vi "Sienar Band - Main Panel.vi"() -> ()   [LabVIEW 2016]
uses:
  <userlib>/LVLibSVM/LibSVM Sparse/Controls/Grid parameters.ctl
  <vilib>/Math Plots/3D Math Plots/3D Surface/3D Surface XCtrl/3D Surface.xctl
  Typedef/SVM predict class.ctl
  Typedef/SVM train class.ctl
  Typedef/SIENAR Band - States.ctl
  <vilib>/BLE/type_def/connection_status_bundle.ctl
  <vilib>/BLE/type_def/address_type.ctl
  Typedef/Event cluster.ctl
  <userlib>/LVLibSVM/LibSVM Dense/Wrapper API/Controls/svmdense_problem.ctl
  <userlib>/LVLibSVM/LibSVM Dense/Wrapper API/Controls/svmdense_model.ctl
  <userlib>/LVLibSVM/LibSVM Sparse/Wrapper API/Controls/svm_parameter.ctl
  <userlib>/LVLibSVM/LibSVM Sparse/Wrapper API/Controls/svm_type.ctl
  <userlib>/LVLibSVM/LibSVM Sparse/Wrapper API/Controls/svm_kernel_type.ctl
  Typedef/BLE char handle.ctl
  <userlib>/LVLibSVM/LibSVM Sparse/Controls/Options Training.ctl
  <userlib>/LVLibSVM/LibSVM Dense/SubVIs/SVM Dense Train C_SVC.vi
  <userlib>/LVLibSVM/LibSVM Dense/Wrapper API/svmdense_predict.vi
  <userlib>/LVLibSVM/Tools/SubVIs/Dense - Scale Problem Linear.vi
  <userlib>/LVLibSVM/LibSVM Dense/Wrapper API/svmdense_train.vi
  <vilib>/Utility/xml.llb/Read From XML File(string).vi
  <vilib>/Utility/xml.llb/Write to XML File(string).vi
panel:
  in  "Show RAW data":bool
  in  "Tab Control":T1(tab)
  in  "Timeout":u16=1000 format="%.0fms"
  in  "Latency":u16 max=500 step=1
  in  "Max interval":u16=50 caption="Connection interval (max)" min=10 max=4000 step=1 format="%.0fms"
  in  "Min interval":u16=20 caption="Connection interval (min)" min=10 max=4000 step=1 format="%.0fms"
  out "Devices":i32(listbox)=-1
  out "BLE Status":bool
  in  "Connect BLE":bool
  in  "Address type":enum8{"Public", "Random"}(ring)
  in  "MAC Address":string="24:0A:C4:04:1C:4E"
  out "BLED112 Dongle Info":string
  in  "Connect dongle":bool
  out "Dongle Status":bool
  in  "USB BLE Dongle port":refnum<visa-resource-name>
  in  "Discover":bool
  in  "Notes":string
  in  "User name":string
  in  "Test label":string
  in  "Open MPU calib":bool
  in  "Acquisition interval":u32=50 min=50 max=1000 step=10 format="%.0fms"
  in  "MPU calib":path=path "C:/Users/Frax/Desktop/Sienar-Band/MPU_calib.ini" caption="Choose MPU calibration file:"
  in  "Confirm settings":bool
  out "Strain chart":T2(graph)
  in  "Open adv viewer":bool
  in  "Stream data":bool
  in  "Clear Plot":bool
  out "YPR chart":cluster{"Yaw":sgl, "Pitch":sgl, "Roll":sgl}(graph)
  in  "Save RAW data":bool
  in  "Open MPU panel":bool
  in  "Save SVM model":bool
  in  "Learn from data":bool
  in  "Split data":bool=TRUE caption="Split data set for cross-validation"
  in  "Load data set":bool
  in  "SVM train Class":T3
  in  "Append data":bool=TRUE caption="Append data to file"
  in  "Save Data set":bool
  in  "Train":bool
  out "Event Going on?":bool
  out "Event Count":u32
  out "Gridsearch result":refnum<class "3D Plot Datatype.lvclass">[](xcontrol)
  in  "Grid parameters":T4={"C start"=-5.0, "Gamma start"=-15.0, "C end"=15.0, "C step"=4.0, "K"=10, "Gamma end"=3.0, "Gamma step"=4.0, "random seed"=-1}
  out "Class detected":T5
  in  "Predict":bool
  in  "Load SVM model":bool
  in  "Exit":bool
  in  "Connection panel":bool
  in  "SVM Analysis panel":bool
  in  "SVM Train panel":bool
  in  "Settings panel":bool
  # "Acquisition settings"
  # "OR"
  # "User settings"
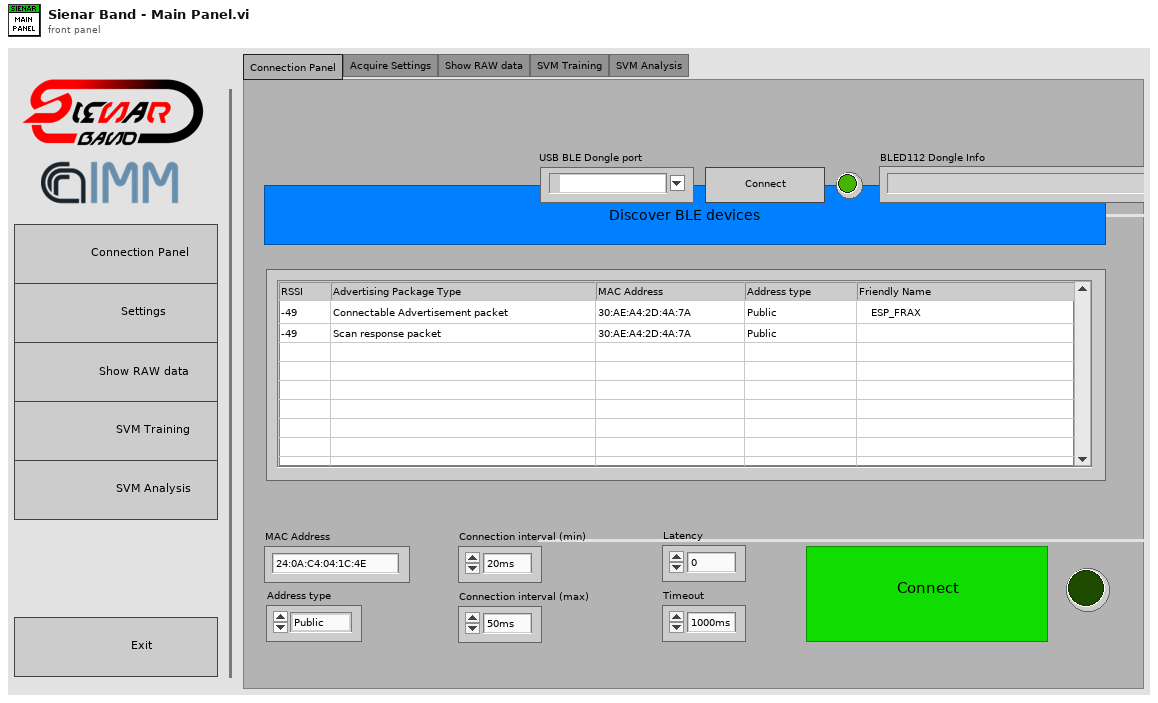
[diagram p1: front panel]
types:
  T1 = enum32{"Connection Panel", "Acquire Settings", "Show RAW data", "SVM Training", "SVM Analysis"}
  T2 = cluster{"Strain sensor 1":sgl, "Strain sensor 2":sgl, "Strain sensor 3":sgl, "Strain sensor 4":sgl, "Strain sensor 5":sgl, "Strain sensor 6":sgl, "Strain sensor 7":sgl, "Strain sensor 8":sgl}
  T3 = typedef "SVM train class.ctl" = enum16{"Grab/Grab release", "Hand flexion/HF release", "Hand extension/HE release", "Tap", "Swipe_CW", "Swipe_CCW"}
  T4 = typedef "Grid parameters.ctl" = cluster{"C start":dbl, "Gamma start":dbl, "C end":dbl, "C step":dbl, "K":i32, "Gamma end":dbl, "Gamma step":dbl, "random seed":i32}
  T5 = typedef "SVM predict class.ctl" = enum16{"Grab", "Grab release", "Hand flexion", "Hand flexion release", "Hand extension", "Hand extension release", "Tap", "Swipe_CW", "Swipe_CCW"}
  T6 = cluster{"Strain data":cluster{"Strain sensor 1":sgl, "Strain sensor 2":sgl, "Strain sensor 3":sgl, "Strain sensor 4":sgl, "Strain sensor 5":sgl, "Strain sensor 6":sgl, "Strain sensor 7":sgl, "Strain sensor 8":sgl}, "YPR data":cluster{"Yaw":sgl, "Pitch":sgl, "Roll":sgl}}
  T7 = typedef "connection_status_bundle.ctl" = cluster{"MAC Address":string, "cnx handle":u8, "cnx flags":u8, "Address Type":T8, "Connection Interval (ms)":u16, "Timeout(ms)":u16, "Latency":u16, "bonding handle":u8}
  T8 = typedef "address_type.ctl" = u8
  T9 = typedef "Event cluster.ctl" = cluster{"Base line":dbl[], "Event data":dbl[][], "Duration":dbl, "Event ongoing":bool, "SVM train Class":T3, "SVM predict Class":T5}
  T10 = typedef "svmdense_problem.ctl" = cluster{"Y":dbl[], "X":cluster{"x":dbl[]}[]}
  T11 = typedef "svmdense_model.ctl" = cluster{"param":T12, "nr_class":i32, "l":i32, "SV":cluster{"Array":dbl[]}[], "sv_coef":dbl[][], "rho":dbl[], "probA":dbl[], "probB":dbl[], "sv_indices":i32[], "label":i32[], "nSV":i32[]}
  T12 = typedef "svm_parameter.ctl" = cluster{"svm_type":T13, "kernel_type":T14, "degree":i32, "gamma":dbl, "coef0":dbl, "cache_size":dbl, "eps":dbl, "C":dbl, "weight_label":i32[], "weight":dbl[], "nu":dbl, "p":dbl, "shrinking":bool, "probability":bool}
  T13 = typedef "svm_type.ctl" = enum32{"C_SVC", "NU_SVC", "ONE_CLASS", "EPSILON_SVR", "NU_SVR"}
  T14 = typedef "svm_kernel_type.ctl" = enum32{"LINEAR", "POLY", "RBF", "SIGMOID", "PRECOMPUTED"}
  T15 = cluster{"Conn Status":T7, "MAC Address":string, "Is Connected":bool, "Handle table":string[][], "channel map":u16, "Event cluster":T9, "Data set":dbl[][], "Dense Problem":T10, "Model":T11}
  T16 = typedef "SIENAR Band - States.ctl" = enum16{"Idle", "Connect Dongle", "Discover BLE", "Connect BLE", "Discover Services", "Disconnect BLE", "Confirm settings", "Open advanced viewer", "Open MPU panel", "Set Stream settings", "Stream data", "Stop stream", "Stop", "Save RAW data", "SVM - Train", "SVM - Check for event", "SVM - Extract features", "SVM - Learn from data", "SVM - Load data set", "SVM - Save data set", "SVM - Load SVM model", "SVM - Save SVM model", "SVM - Start predict", "Exit"}
  T17 = typedef "Options Training.ctl" = cluster{"cache_size":dbl, "eps":dbl, "shrinking":bool, "probability":bool}
  T18 = enum16{"open", "replace", "create", "open or create", "replace or create", "replace or create with confirmation"}
  T19 = typedef "BLE char handle.ctl" = u16
  T20 = cluster{"Avg Strain data out":cluster{"Strain sensor 1":sgl, "Strain sensor 2":sgl, "Strain sensor 3":sgl, "Strain sensor 4":sgl, "Strain sensor 5":sgl, "Strain sensor 6":sgl, "Strain sensor 7":sgl, "Strain sensor 8":sgl}, "YPR data":cluster{"Yaw":sgl, "Pitch":sgl, "Roll":sgl}}
  T21 = cluster{"Strain sensor 1":sgl, "Strain sensor 2":sgl, "Strain sensor 3":sgl, "Strain sensor 4":sgl, "Strain sensor 5":sgl, "Strain sensor 6":sgl, "Strain sensor 7":sgl, "Strain sensor 8":sgl}[]
  T22 = typedef "Kernel.ctl" = cluster{"Type":T14, "Degree":i32, "Gamma":dbl, "Coef0":dbl}
  T23 = typedef "Parameters C_SVC.ctl" = cluster{"C":dbl, "weight_label":i32[], "weight":dbl[]}
  T24 = cluster{"libsvm options":T17, "libsvm weights":T23}
  T25 = typedef "svm_problem.ctl" = cluster{"y":dbl[], "x":cluster{T26[]}[]}
  T26 = typedef "svm_node.ctl" = cluster{"index":i32, "value":dbl}
  T27 = cluster{"Strain sensor 1":dbl, "Strain sensor 2":dbl, "Strain sensor 3":dbl, "Strain sensor 4":dbl, "Strain sensor 5":dbl, "Strain sensor 6":dbl, "Strain sensor 7":dbl, "Strain sensor 8":dbl}[]
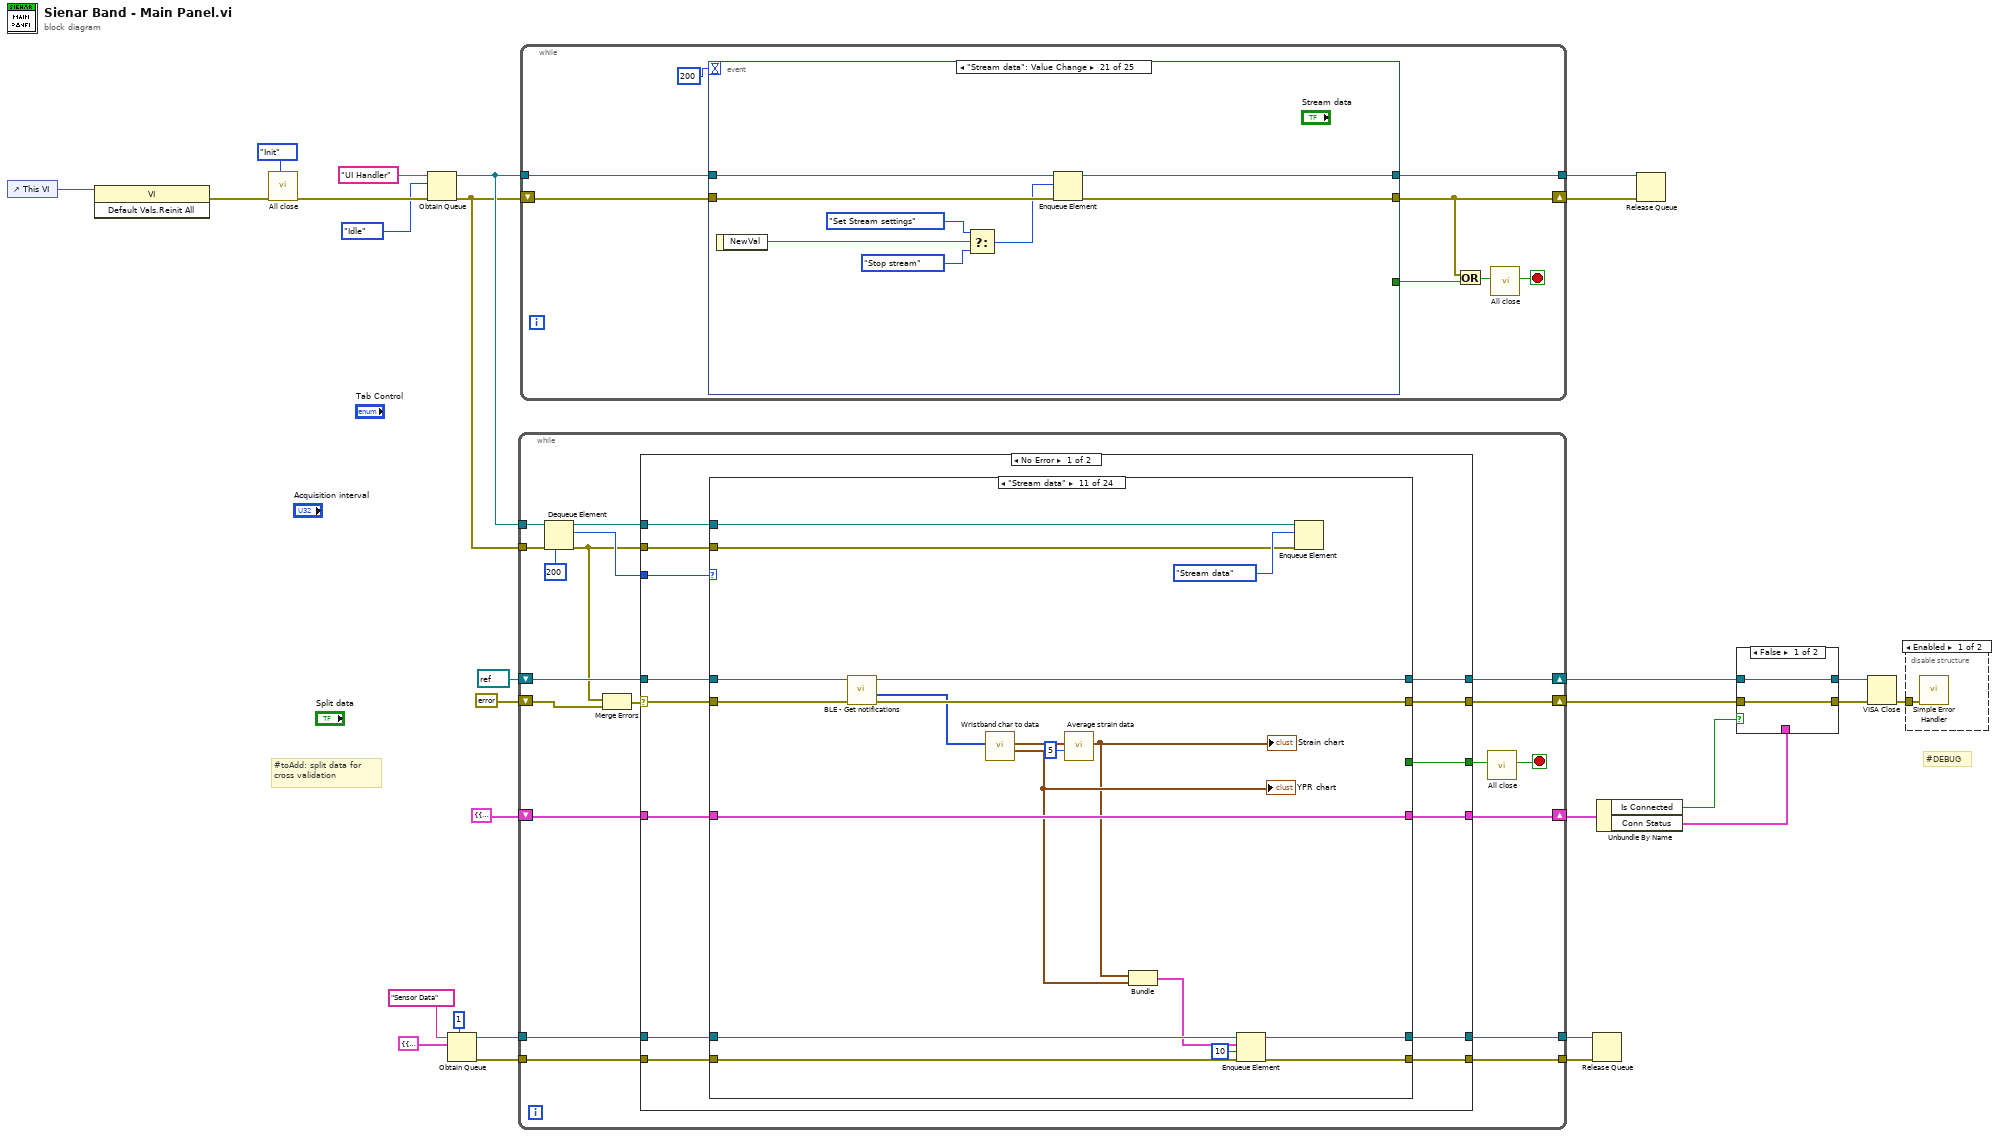
[diagram p0: block diagram]
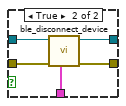
[diagram p3: hidden frame]
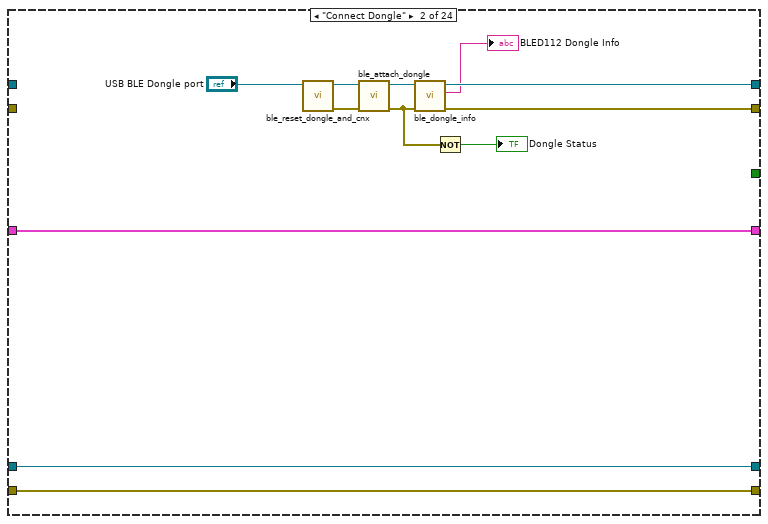
[diagram p5: hidden frame]
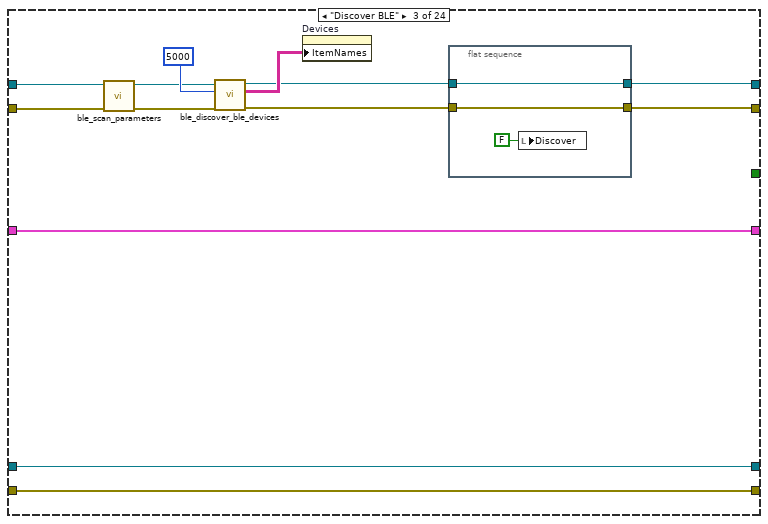
[diagram p6: hidden frame]
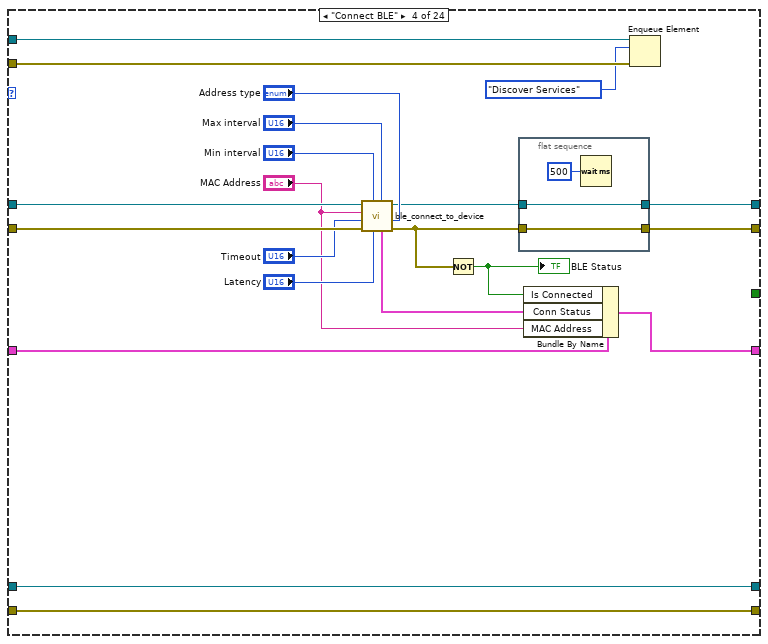
[diagram p7: hidden frame]
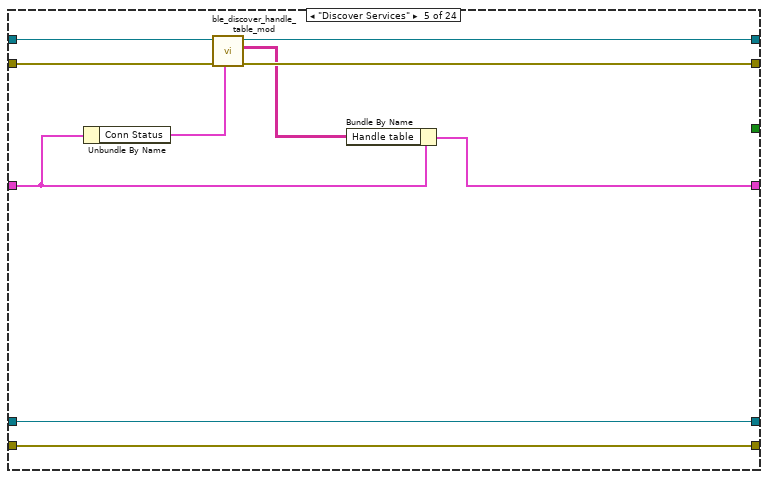
[diagram p8: hidden frame]
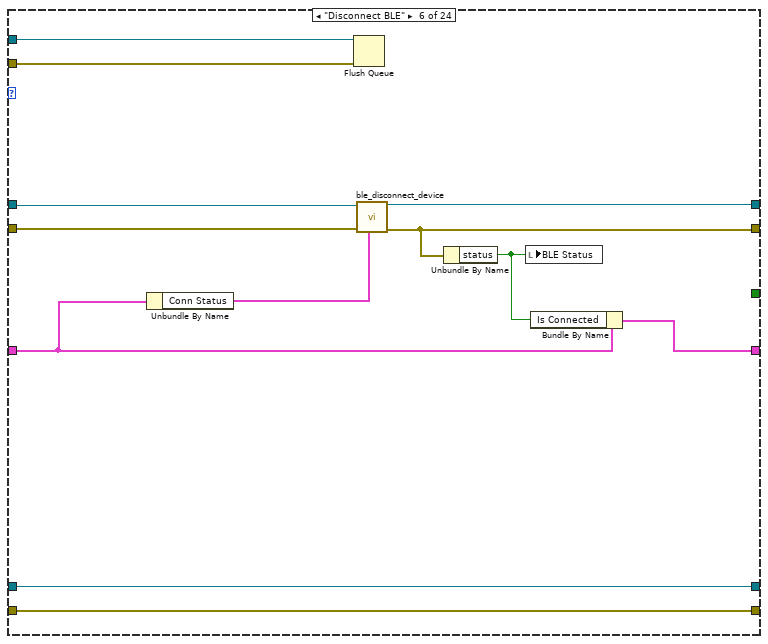
[diagram p9: hidden frame]
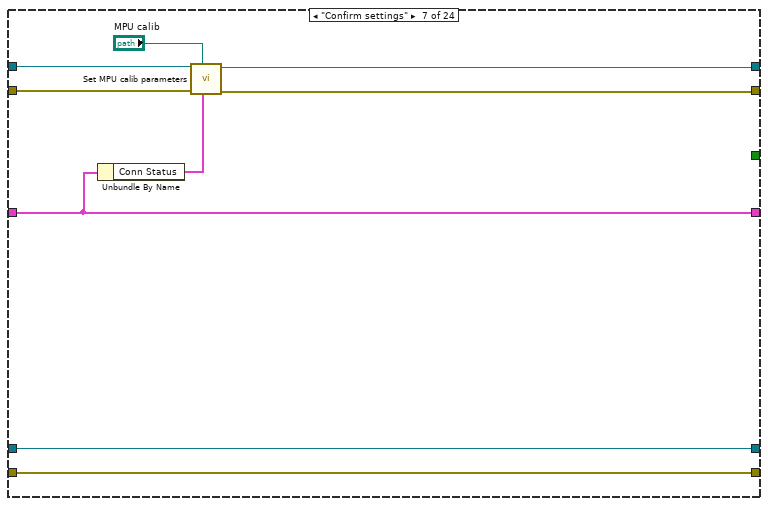
[diagram p10: hidden frame]
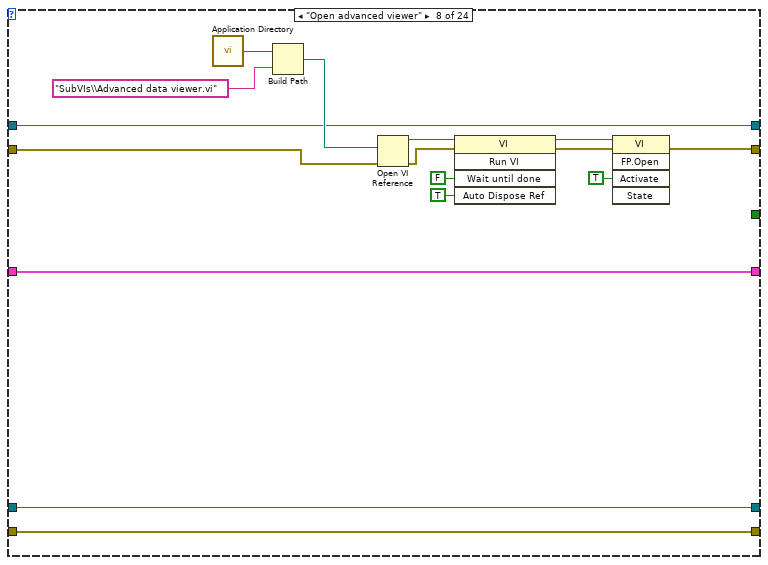
[diagram p11: hidden frame]
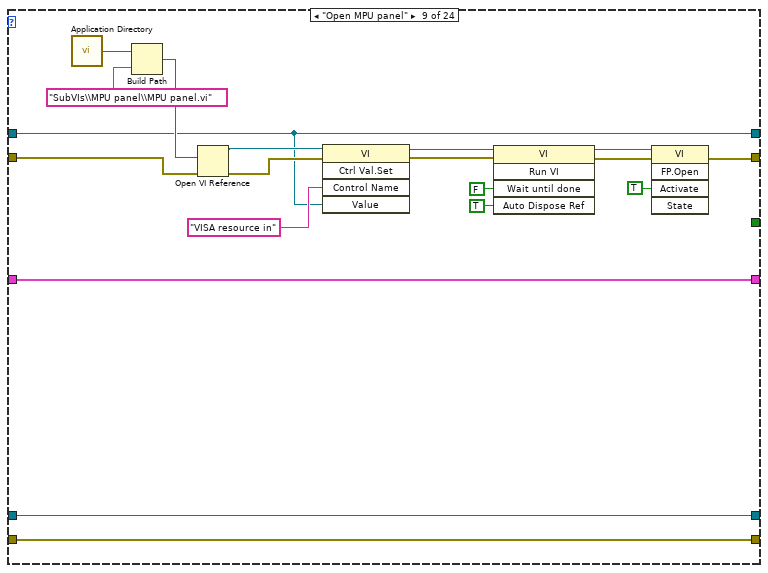
[diagram p12: hidden frame]
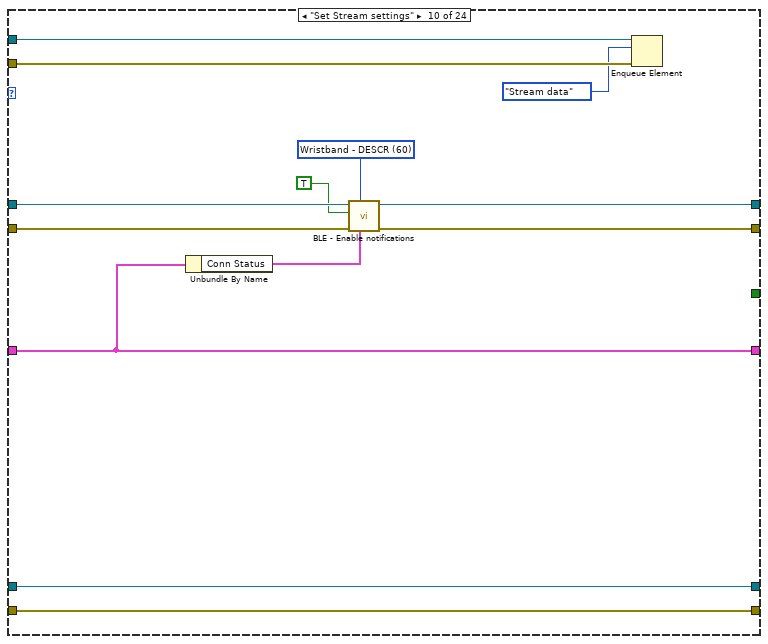
[diagram p13: hidden frame]
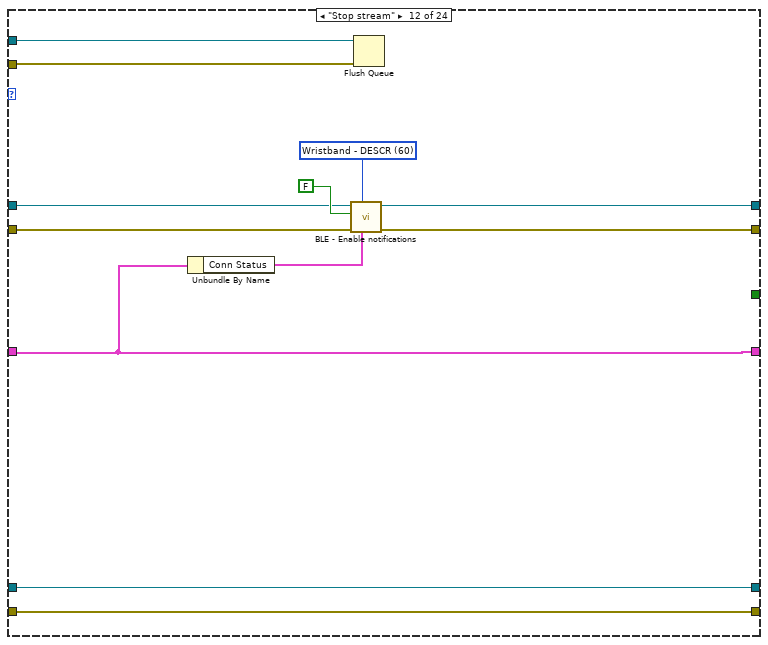
[diagram p14: hidden frame]
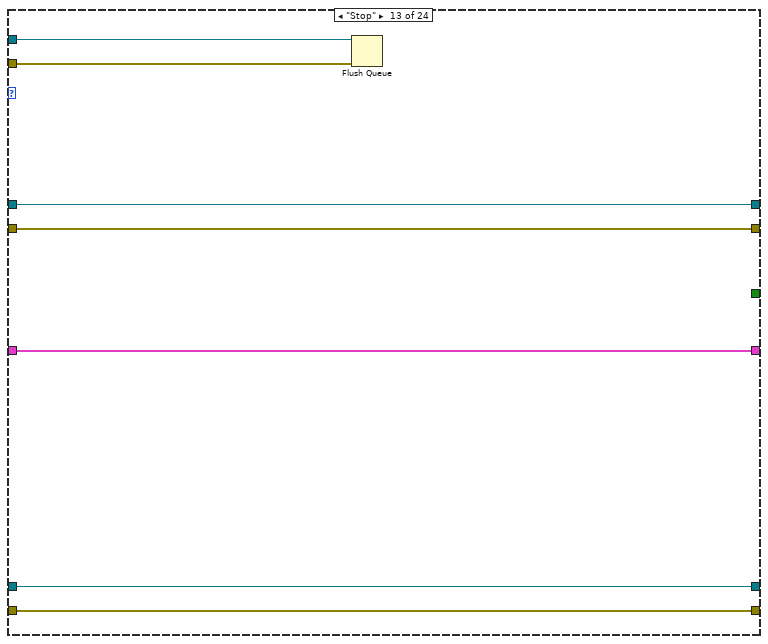
[diagram p15: hidden frame]
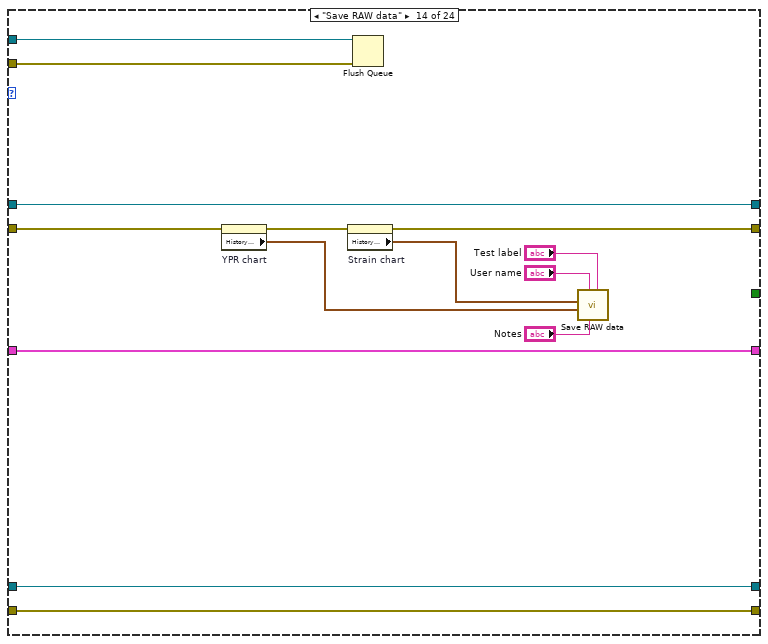
[diagram p16: hidden frame]
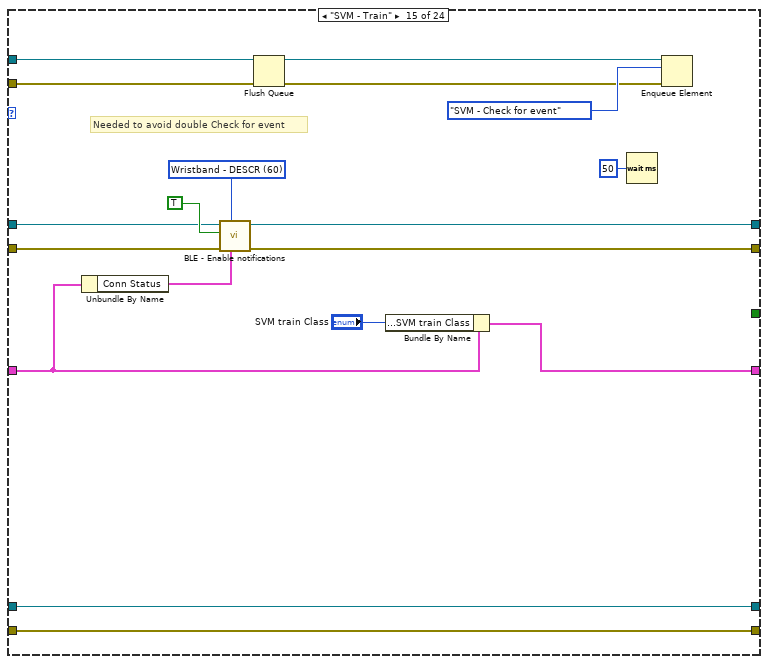
[diagram p17: hidden frame]
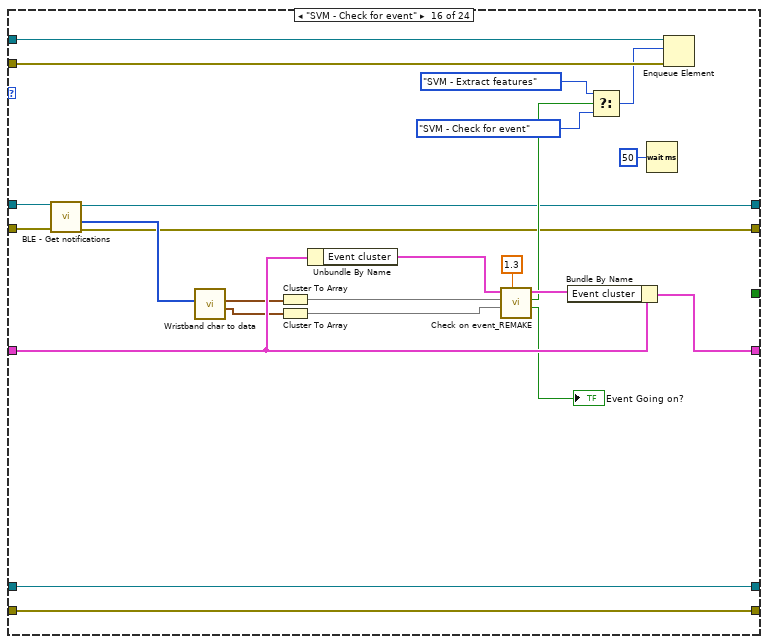
[diagram p18: hidden frame]
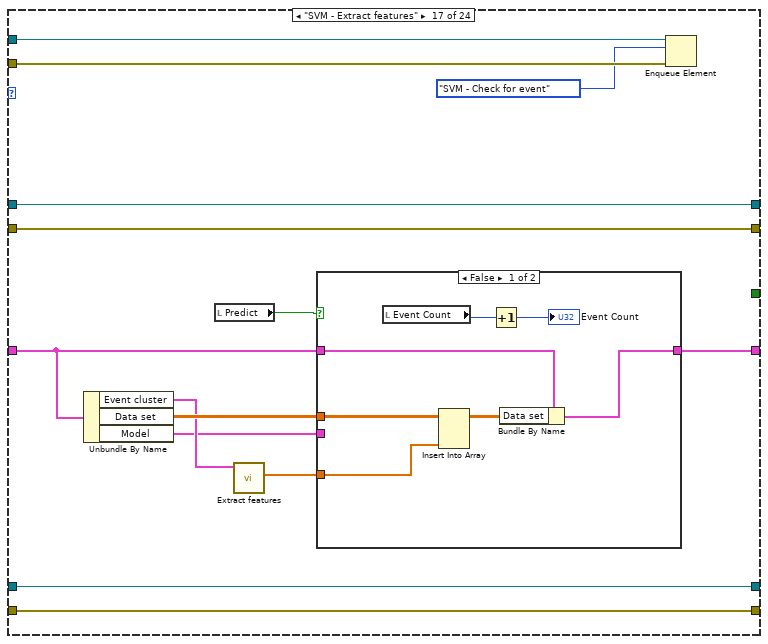
[diagram p19: hidden frame]
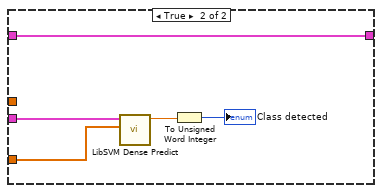
[diagram p20: hidden frame]
diagram:
  # "#toAdd: split data for\ncross validation"
  # "#DEBUG"
  n1 = control-ref of="This VI"() -> (w23:refnum<vi>)
  n2 = invoke class="VI" method="Default Vals.Reinit All"(reference=w23) -> (error out=w22:errorcluster)  [unwired: 2 in, 2 out]
  n3 = call "All close.vi"("Operation (Check)"=enum16{"Init", "Check"}."Init", "Error In"=w22) -> ("Error Out"=w25:errorcluster)  [unwired: 8 in, 1 out]
  n4 = Obtain Queue(name (unnamed)="UI Handler", element data type=SIENAR_Band_-_States."Idle", error in (no error)=w25) -> (queue out=w21:refnum<queue>, error out=w20:errorcluster)  [unwired: 2 in, 1 out]
  n5 = Obtain Queue(max queue size (-1, unlimited)=1, name (unnamed)="Sensor Data", element data type=T6 {"Strain data"={"Strain sensor 1"=0.0, "Strain sensor 2"=0.0, "Strain sensor 3"=0.0, "Strain sensor 4"=0.0, "Strain sensor 5"=0.0, "Strain sensor 6"=0.0, "Strain sensor 7"=0.0, "Strain sensor 8"=0.0}, "YPR data"={"Yaw"=0.0, "Pitch"=0.0, "Roll"=0.0}} ("Wristband data")) -> (queue out=w7:refnum<queue>, error out=w6:errorcluster)  [unwired: 2 in, 1 out]
  n6 = while {
    tunnel: w21 -> [w47]
    tunnel: w20 -> [w46]
    shift-right: [w40] -> w12
    shift-left: errorcluster {"status"=FALSE, "code"=0, "source"=""} ("error out") -> [w36]
    shift-right: [w42] -> w11
    shift-left: refnum<visa-resource-name> refnum ("COM Bluegiga out") -> [w41]
    shift-right: [w39] -> w10
    shift-left: T15 {"Conn Status"={"MAC Address"="", "cnx handle"=0, "cnx flags"=0, "Address Type"=125, "Connection Interval (ms)"=125, "Timeout(ms)"=125, "Latency"=0, "bonding handle"=0}, "MAC Address"="", "Is Connected"=FALSE, "Handle table"=[], "channel map"=32767, "Event cluster"={"Base line"=[], "Event data"=[], "Duration"=0.0, "Event ongoing"=FALSE, "SVM train Class"=enum."Grab/Grab release", "SVM predict Class"=enum."Grab"}, "Data set"=[], "Dense Problem"={"Y"=[], "X"=[]}, "Model"={"param"={"svm_type"=enum."C_SVC", "kernel_type"=enum."LINEAR", "degree"=0, "gamma"=0.0, "coef0"=0.0, "cache_size"=0.0, "eps"=0.0, "C"=0.0, "weight_label"=[], "weight"=[], "nu"=0.0, "p"=0.0, "shrinking"=FALSE, "probability"=FALSE}, "nr_class"=0, "l"=0, "SV"=[], "sv_coef"=[], "rho"=[], "probA"=[], "probB"=[], "sv_indices"=[], "label"=[], "nSV"=[]}} ("Cluster") -> [w38]
    tunnel: w7 -> [w32]
    tunnel: w6 -> [w31]
    tunnel: [w30] -> w5
    tunnel: [w29] -> w4
    stop <- w45 stop-if-true
    n7 = Dequeue Element(queue=w47, timeout in ms (-1)=200, error in (no error)=w46) -> (queue out=w43:refnum<queue>, element=w44:T16, error out=w35:errorcluster)  [unwired: 1 out]
    n8 = Merge Errors(w35, w36) -> (w37:errorcluster)
    n9 = case shown="No Error" w37 {
      selector: w37 -> [w52 w419]
      tunnel: w44 -> [w61 _]
      tunnel: w43 -> [w60 _]
      tunnel: w35 -> [w59 _]
      tunnel: [w58 w420] -> w34
      tunnel: [w57 w416] -> w42
      tunnel: w41 -> [w56 w417]
      tunnel: [w55 w418] -> w40
      tunnel: [w54 w415] -> w39
      tunnel: w38 -> [w53 w415]
      tunnel: w32 -> [w51 w414]
      tunnel: w31 -> [w50 w413]
      tunnel: [w49 w414] -> w30
      tunnel: [w48 w413] -> w29
      frame No Error {
        n10 = case shown="\"Stream data\"" w61 {
          tunnel: w60 -> [_ _ _ w108 _ w137 _ _ _ w197 w211 w228 w232 w247 w261 w288 w296 _ _ _ w374 _ _ _]
          tunnel: w59 -> [_ _ _ w107 _ w136 _ _ _ w196 w210 w227 w231 w246 w262 w289 w295 _ _ _ w375 _ _ _]
          tunnel: [_ _ _ _ _ _ _ _ _ _ _ _ _ _ _ _ _ _ _ _ _ TRUE _ _] -> w58
          tunnel: [w66 w77 w83 w95 w125 w138 w143 w153 w169 w190 w213 w219 w234 w249 w252 w274 w303 w336 w346 w361 w376 w394 w405 w412] -> w57
          tunnel: [w65 w76 w82 w98 w126 w134 w142 w151 w168 w189 w214 w220 w235 w243 w251 w273 w302 w322 w338 w350 w377 w393 w404 w411] -> w55
          tunnel: w56 -> [w66 _ w88 w115 w128 w140 w146 w153 w169 w191 w216 w223 w234 w249 w255 w276 w303 w336 w346 w361 w380 w394 w405 w412]
          tunnel: w52 -> [w65 _ w87 w114 w127 w139 w147 w152 w173 w192 w215 w222 w235 w245 w254 w275 w302 w323 w339 w349 w379 w393 w404 w411]
          tunnel: [w62 w75 w81 w104 w121 w131 w141 w165 w184 w186 w209 w221 w233 w248 w265 w286 w301 w319 w337 w358 w378 w395 w400 w408] -> w54
          tunnel: w53 -> [w62 w75 w81 w105 w122 w133 w141 w165 w184 w186 w209 w221 w233 w248 w253 w287 w300 w320 w341 w359 w378 w395 w401 w408]
          tunnel: w51 -> [w64 w74 w80 w100 w120 w130 w149 w163 w183 w194 w208 w218 w230 w240 w267 w291 w305 w325 w345 w356 w389 w391 w403 w410]
          tunnel: w50 -> [w63 w73 w79 w99 w119 w129 w148 w164 w182 w193 w207 w217 w229 w239 w266 w290 w304 w324 w344 w355 w388 w390 w402 w409]
          tunnel: [w64 w74 w80 w100 w120 w130 w149 w163 w183 w194 w206 w218 w230 w240 w267 w291 w305 w325 w345 w356 w389 w391 w403 w410] -> w49
          tunnel: [w63 w73 w79 w99 w119 w129 w148 w164 w182 w193 w205 w217 w229 w239 w266 w290 w304 w324 w344 w355 w388 w390 w402 w409] -> w48
          frame "Idle" {
          }
          frame "Connect Dongle" {
            n11 = call <vilib>:"ble_reset_dongle_and_cnx.vi"("COM Bluegiga in"="USB BLE Dongle port") -> ("error out"=w72:errorcluster, "COM Bluegiga out"=w71:refnum<visa-resource-name>)  [unwired: 9 in]
            n12 = call <vilib>:"ble_attach_dongle.vi"("error in (no error)"=w72, "COM Bluegiga in"=w71) -> ("error out"=w69:errorcluster, "COM Bluegiga out"=w70:refnum<visa-resource-name>)  [unwired: 8 in]
            n13 = call <vilib>:"ble_dongle_info.vi"("error in (no error)"=w69, "COM Bluegiga in"=w70) -> ("error out"=w76:errorcluster, "info"=→"BLED112 Dongle Info":string, "COM Bluegiga out"=w77:refnum<visa-resource-name>)  [unwired: 7 in]
            n14 = Not(x=w69) -> (.not. x?=→"Dongle Status":bool)
          }
          frame "Discover BLE" {
            n15 = call <vilib>:"ble_scan_parameters.vi"("error in (no error)"=w87, "COM Bluegiga in"=w88) -> ("error out"=w90:errorcluster, "COM Bluegiga out"=w89:refnum<visa-resource-name>)  [unwired: 7 in, 1 out]
            n16 = call <vilib>:"ble_discover_ble_devices.vi"("error in (no error)"=w90, "Scan Duration (10000ms)"=u32 5000, "COM Bluegiga in"=w89) -> ("error out"=w84:errorcluster, "Devices"=w86:string[][], "COM Bluegiga out"=w85:refnum<visa-resource-name>)  [unwired: 6 in]
            n17 = property on="Devices" class="MCListbox (strict)"("ItemNames"=w86) -> ()  [unwired: 2 in, 2 out]
            n18 = flat-sequence {
              tunnel: w85 -> [w94]
              tunnel: w84 -> [w93]
              tunnel: [w94] -> w83
              tunnel: [w93] -> w82
              frame #0 {
                n19 = local write "Discover"(FALSE ("Discover")) -> ()
              }
            }
          }
          frame "Connect BLE" {
            n20 = call <vilib>:"ble_connect_to_device.vi"("Address Type"="Address type", "Connection Interval Max (95ms)"="Max interval", "Latency(0)"="Latency", "Connection Interval Min (75ms)"="Min interval", "error in (no error)"=w114, "Timeout(1000ms)"="Timeout", "MAC Address"="MAC Address", "COM Bluegiga in"=w115) -> ("error out"=w97:errorcluster, "COM Bluegiga out"=w96:refnum<visa-resource-name>, "Connection Status"=w103:T7)  [unwired: 1 in]
            n21 = Not(x=w97) -> (.not. x?=w101:bool)
            "BLE Status" <- w101
            n22 = flat-sequence {
              tunnel: [w117] -> w98
              tunnel: w97 -> [w117]
              tunnel: w96 -> [w116]
              tunnel: [w116] -> w95
              frame #0 {
                n23 = Wait (ms)(milliseconds to wait=u32 500) -> ()  [unwired: 1 out]
              }
            }
            n24 = Bundle By Name(cluster=w105, "Is Connected"=w101, "Conn Status"=w103, "MAC Address"="MAC Address") -> (w104:T15)
            n25 = Enqueue Element(queue=w108, element=SIENAR_Band_-_States."Discover Services", error in (no error)=w107) -> ()  [unwired: 1 in, 3 out]
          }
          frame "Discover Services" {
            n26 = Unbundle By Name(w122) -> ("Conn Status"=w124:T7)
            n27 = call "ble_discover_handle_table_mod.vi"("Connection Status"=w124, "error in (no error)"=w127, "COM Bluegiga in"=w128) -> ("error out"=w126:errorcluster, "Handle table"=w123:string[][], "COM Bluegiga out"=w125:refnum<visa-resource-name>)  [unwired: 5 in, 1 out]
            n28 = Bundle By Name(cluster=w122, "Handle table"=w123) -> (w121:T15)
          }
          frame "Disconnect BLE" {
            n29 = Unbundle By Name(w133) -> ("Conn Status"=w135:T7)
            n30 = Flush Queue(queue=w137, error in (no error)=w136) -> ()  [unwired: 3 out]
            n31 = call <vilib>:"ble_disconnect_device.vi"("Connection Status"=w135, "error in (no error)"=w139, "COM Bluegiga in"=w140) -> ("error out"=w134:errorcluster, "COM Bluegiga out"=w138:refnum<visa-resource-name>)  [unwired: 7 in]
            n32 = Unbundle By Name(w134) -> ("status"=w132:bool)
            n33 = local write "BLE Status"(w132) -> ()
            n34 = Bundle By Name(cluster=w133, "Is Connected"=w132) -> (w131:T15)
          }
          frame "Confirm settings" {
            n35 = Unbundle By Name(w141) -> ("Conn Status"=w144:T7)
            n36 = call "Set MPU calib parameters.vi"("Connection Status"=w144, "Calib file path"="MPU calib", "Error In"=w147, "VISA resource in"=w146) -> ("Error Out"=w142:errorcluster, "VISA resource out"=w143:refnum<visa-resource-name>)  [unwired: 6 in]
          }
          frame "Open advanced viewer" {
            n37 = call <vilib>:"Application Directory.vi"() -> ("Application Directory"=w157:path)
            n38 = Build Path(base path=w157, name or relative path="SubVIs\\Advanced data viewer.vi") -> (appended path=w156:path)
            n39 = Open VI Reference(vi path=w156, error in (no error)=w152) -> (vi reference=w154:refnum<vi>, error out=w150:errorcluster)  [unwired: 4 in]
            n40 = invoke class="VI" method="Run VI"(reference=w154, error in=w150, "Wait until done"=FALSE ("Wait Until Done"), "Auto Dispose Ref"=TRUE ("Auto Dispose Reference")) -> (reference out=w160:refnum<vi>, error out=w159:errorcluster)  [unwired: 1 in, 3 out]
            n41 = invoke class="VI" method="FP.Open"(reference=w160, error in=w159, "Activate"=TRUE ("Activate?")) -> (error out=w151:errorcluster)  [unwired: 2 in, 4 out]
          }
          frame "Open MPU panel" {
            n42 = call <vilib>:"Application Directory.vi"() -> ("Application Directory"=w176:path)
            n43 = Build Path(base path=w176, name or relative path="SubVIs\\MPU panel\\MPU panel.vi") -> (appended path=w175:path)
            n44 = Open VI Reference(vi path=w175, error in (no error)=w173) -> (vi reference=w171:refnum<vi>, error out=w170:errorcluster)  [unwired: 4 in]
            n45 = invoke class="VI" method="Ctrl Val.Set"(reference=w171, error in=w170, "Control Name"="VISA resource in", "Value"=w169) -> (reference out=w167:refnum<vi>, error out=w166:errorcluster)  [unwired: 1 in, 3 out]
            n46 = invoke class="VI" method="Run VI"(reference=w167, error in=w166, "Wait until done"=FALSE ("Wait Until Done"), "Auto Dispose Ref"=TRUE ("Auto Dispose Reference")) -> (reference out=w179:refnum<vi>, error out=w178:errorcluster)  [unwired: 1 in, 3 out]
            n47 = invoke class="VI" method="FP.Open"(reference=w179, error in=w178, "Activate"=TRUE ("Activate?")) -> (error out=w168:errorcluster)  [unwired: 2 in, 4 out]
          }
          frame "Set Stream settings" {
            w187 = T19 60 items=["MPU data"=42, "MPU data - DESCR"=43, "Accel calib parameters"=45, "Gyro calib parameters"=47, "Mag calib parameters - 1"=49, "Mag calib parameters - 2"=51, "YPR"=53, "YPR - DESCR"=54, "Strain sensors"=56, "Strain sensors - DESCR"=57, "Wristband"=59, "Wristband - DESCR"=60] ("BLE char handle")
            n48 = Unbundle By Name(w186) -> ("Conn Status"=w185:T7)
            n49 = call "BLE - Enable notifications.vi"("Conn Status"=w185, "Descriptor handle"=w187, "Error In"=w192, "Enable notifications"=TRUE, "COM Bluegiga in"=w191) -> ("Error Out"=w189:errorcluster, "COM Bluegiga out"=w190:refnum<visa-resource-name>)  [unwired: 5 in]
            n50 = Enqueue Element(queue=w197, element=SIENAR_Band_-_States."Stream data", error in (no error)=w196) -> ()  [unwired: 1 in, 3 out]
          }
          frame "Stream data" {
            n51 = call "BLE - Get notifications.vi"("COM Bluegiga in"=w216, "Error In"=w215) -> ("COM Bluegiga out"=w213:refnum<visa-resource-name>, "Notified Data"=w204:u8[], "Error Out"=w214:errorcluster)  [unwired: 5 in, 1 out]
            n52 = call "Wristband char to data.vi"("Wristband char value"=w204) -> ("YPR data"=w201:cluster{"Yaw":sgl, "Pitch":sgl, "Roll":sgl}, "Strain data"=w200:T2)  [unwired: 8 in, 1 out]
            "YPR chart" <- w201
            n53 = call "Average strain data.vi"("Window points"=5, "Strain data in"=w200) -> ("Avg Strain data out"=w199:T2)  [unwired: 8 in, 1 out]
            "Strain chart" <- w199
            n54 = Bundle("Avg Strain data out"=w199, "YPR data"=w201) -> (w203:T20)  [unwired: 1 in]
            n55 = Enqueue Element(queue=w208, element=w203, timeout in ms (-1)=10, error in (no error)=w207) -> (queue out=w206:refnum<queue>, error out=w205:errorcluster)  [unwired: 1 out]
            n56 = Enqueue Element(queue=w211, element=SIENAR_Band_-_States."Stream data", error in (no error)=w210) -> ()  [unwired: 1 in, 3 out]
          }
          frame "Stop stream" {
            w225 = T19 60 items=["MPU data"=42, "MPU data - DESCR"=43, "Accel calib parameters"=45, "Gyro calib parameters"=47, "Mag calib parameters - 1"=49, "Mag calib parameters - 2"=51, "YPR"=53, "YPR - DESCR"=54, "Strain sensors"=56, "Strain sensors - DESCR"=57, "Wristband"=59, "Wristband - DESCR"=60] ("BLE char handle")
            n57 = Unbundle By Name(w221) -> ("Conn Status"=w224:T7)
            n58 = call "BLE - Enable notifications.vi"("Conn Status"=w224, "Descriptor handle"=w225, "Error In"=w222, "Enable notifications"=FALSE, "COM Bluegiga in"=w223) -> ("Error Out"=w220:errorcluster, "COM Bluegiga out"=w219:refnum<visa-resource-name>)  [unwired: 5 in]
            n59 = Flush Queue(queue=w228, error in (no error)=w227) -> ()  [unwired: 3 out]
          }
          frame "Stop" {
            n60 = Flush Queue(queue=w232, error in (no error)=w231) -> ()  [unwired: 3 out]
          }
          frame "Save RAW data" {
            n61 = property on="YPR chart" class="WFChart (strict)"(error in=w245) -> (error out=w244:errorcluster, "History Data"=w237:cluster{"Yaw":sgl, "Pitch":sgl, "Roll":sgl}[])  [unwired: 1 in, 1 out]
            n62 = property on="Strain chart" class="WFChart (strict)"(error in=w244) -> (error out=w243:errorcluster, "History Data"=w238:T21)  [unwired: 1 in, 1 out]
            n63 = Flush Queue(queue=w247, error in (no error)=w246) -> ()  [unwired: 3 out]
            n64 = call "Save RAW data.vi"("Test label"="Test label", "Notes"="Notes", "User"="User name", "YPR data"=w237, "Strain data"=w238) -> ()  [unwired: 6 in, 1 out]
          }
          frame "SVM - Train" {
            w257 = T19 60 items=["MPU data"=42, "MPU data - DESCR"=43, "Accel calib parameters"=45, "Gyro calib parameters"=47, "Mag calib parameters - 1"=49, "Mag calib parameters - 2"=51, "YPR"=53, "YPR - DESCR"=54, "Strain sensors"=56, "Strain sensors - DESCR"=57, "Wristband"=59, "Wristband - DESCR"=60] ("BLE char handle")
            # "Needed to avoid double Check for event"
            n65 = Unbundle By Name(w253) -> ("Conn Status"=w256:T7)
            n66 = call "BLE - Enable notifications.vi"("Conn Status"=w256, "Descriptor handle"=w257, "Error In"=w254, "Enable notifications"=TRUE, "COM Bluegiga in"=w255) -> ("Error Out"=w251:errorcluster, "COM Bluegiga out"=w252:refnum<visa-resource-name>)  [unwired: 5 in]
            n67 = Flush Queue(queue=w261, error in (no error)=w262) -> (queue out=w260:refnum<queue>, error out=w259:errorcluster)  [unwired: 1 out]
            n68 = Bundle By Name(cluster=w253, "Event cluster.SVM train Class"="SVM train Class") -> (w265:T15)
            n69 = Wait (ms)(milliseconds to wait=u32 50) -> ()  [unwired: 1 out]
            n70 = Enqueue Element(queue=w260, element=SIENAR_Band_-_States."SVM - Check for event", error in (no error)=w259) -> ()  [unwired: 1 in, 3 out]
          }
          frame "SVM - Check for event" {
            n71 = call "BLE - Get notifications.vi"("COM Bluegiga in"=w276, "Error In"=w275) -> ("COM Bluegiga out"=w274:refnum<visa-resource-name>, "Notified Data"=w277:u8[], "Error Out"=w273:errorcluster)  [unwired: 5 in, 1 out]
            n72 = call "Wristband char to data.vi"("Wristband char value"=w277) -> ("YPR data"=w270:cluster{"Yaw":sgl, "Pitch":sgl, "Roll":sgl}, "Strain data"=w272:T2)  [unwired: 8 in, 1 out]
            n73 = Cluster To Array(cluster=w272) -> (array=w271:sgl[])
            n74 = Cluster To Array(cluster=w270) -> (array=w269:sgl[])
            n75 = Unbundle By Name(w287) -> ("Event cluster"=w281:T9)
            n76 = call "Check on event_REMAKE.vi"("Derivative Threshold"=1.3, "YPR data"=w269, "Strain data"=w271, "Event cluster in"=w281) -> ("event ongoing"=→"Event Going on?":bool, "new event finished"=w279:bool, "Event cluster"=w280:T9)  [unwired: 4 in, 1 out]
            n77 = Bundle By Name(cluster=w287, "Event cluster"=w280) -> (w286:T15)
            n78 = Select(t=SIENAR_Band_-_States."SVM - Extract features" ("element"), s=w279, f=SIENAR_Band_-_States."SVM - Check for event") -> (s? t:f=w283:T16)
            n79 = Wait (ms)(milliseconds to wait=u32 50) -> ()  [unwired: 1 out]
            n80 = Enqueue Element(queue=w288, element=w283, error in (no error)=w289) -> ()  [unwired: 1 in, 3 out]
          }
          frame "SVM - Extract features" {
            n81 = Unbundle By Name(w300) -> ("Event cluster"=w297:T9, "Data set"=w299:dbl[][], "Model"=w292:T11)
            n82 = local read "Predict"() -> (w293:bool)
            n83 = call "Extract features.vi"("Event cluster"=w297) -> ("Event features"=w298:dbl[])  [unwired: 9 in, 1 out]
            n84 = case shown="False" w293 {
              tunnel: [w312 w317] -> w301
              tunnel: w300 -> [w311 w317]
              tunnel: w299 -> [w310 _]
              tunnel: w298 -> [w308 w316]
              tunnel: w292 -> [_ w315]
              frame False {
                n85 = local read "Event Count"() -> (w307:u32)
                n86 = Insert Into Array(array=w310, new element=w308) -> (w309:dbl[][])  [unwired: 2 in]
                n87 = Increment(x=w307) -> (x+1=→"Event Count":u32)
                n88 = Bundle By Name(cluster=w311, "Data set"=w309) -> (w312:T15)
              }
              frame True {
                n89 = call-poly <userlib>:"LibSVM Dense Predict.vi"("x"=w316, "Model"=w315) -> ("Predicted label"=w314:dbl)  [unwired: 8 in, 1 out]
                n90 = To Unsigned Word Integer(number=w314) -> (unsigned 16bit integer=→"Class detected":u16)
              }
            }
            n91 = Enqueue Element(queue=w296, element=SIENAR_Band_-_States."SVM - Check for event", error in (no error)=w295) -> ()  [unwired: 1 in, 3 out]
          }
          frame "SVM - Learn from data" {
            n92 = Unbundle By Name(w320) -> ("Dense Problem"=w321:T10)
            n93 = call-poly <userlib>:"Scale Linear.vi"("error in (no error)"=w323, "X Scaling limits"=cluster{"X lower":dbl, "X upper":dbl} {"X lower"=0.0, "X upper"=1.0}, "Problem"=w321) -> ("error out"=w332:errorcluster, "Scaled problem"=w326:T10)  [unwired: 6 in, 1 out]
            n94 = call "Kernel grid search.vi"("Error In"=w332, "Grid parameters"="Grid parameters", "Problem"=w326) -> ("Error Out"=w329:errorcluster, "Kernel"=w330:T22, "libsvm"=w328:T24, "3D Surface Plot"=→"Gridsearch result":refnum<class "3D Plot Datatype.lvclass">[])  [unwired: 4 in, 1 out]
            n95 = Unbundle By Name(w328) -> ("libsvm weights"=w327:T23)
            n96 = call-poly <userlib>:"LibSVM Dense Train.vi"("Options"=T17 {"cache_size"=500.0, "eps"=0.001, "shrinking"=TRUE, "probability"=FALSE}, "error in (no error)"=w329, "Param C_SVC"=w327, "Kernel"=w330, "Dense problem"=w326) -> ("error out"=w322:errorcluster, "Model"=w318:T11)  [unwired: 5 in]
            n97 = Bundle By Name(cluster=w320, "Model"=w318) -> (w319:T15)
          }
          frame "SVM - Load data set" {
            n98 = call <userlib>:"Read Problem.vi"("error in (no error)"=w339) -> ("error out"=w342:errorcluster, "svm_problem"=w343:T25)  [unwired: 9 in]
            n99 = call <userlib>:"Sparse To Dense Problem.vi"("error in (no error)"=w342, "Sparse Problem"=w343) -> ("error out"=w338:errorcluster, "Dense Problem"=w340:T10)  [unwired: 8 in]
            n100 = Bundle By Name(cluster=w341, "Dense Problem"=w340) -> (w337:T15)
          }
          frame "SVM - Save data set" {
            # "#debug per il salvataggio\nsu disco!!!! Probabilmente conviene\nsalvare direttamente l'array 2D"
            # "Reset data set once is saved"
            n101 = case shown="True" "Append data" {
              tunnel: [w363 w373] -> w354
              tunnel: [w362 w372] -> w353
              tunnel: w349 -> [w364 w366]
              frame False {
                n102 = Open/Create/Replace File(error in=w364, operation (0:open)=T18."create") -> (refnum out=w362:refnum<file>, error out=w363:errorcluster)  [unwired: 4 in, 1 out]
              }
              frame True {
                n103 = Open/Create/Replace File(error in=w366, operation (0:open)=T18."open or create") -> (refnum out=w370:refnum<file>, error out=w369:errorcluster)  [unwired: 4 in, 1 out]
                n104 = Set File Position(offset (in bytes) (0)=i64 0, refnum=w370, from (0:start)=enum16{"start", "end", "current"}."end", error in=w369) -> (refnum out=w372:refnum<file>, error out=w373:errorcluster)
              }
            }
            n105 = Unbundle By Name(w359) -> ("Data set"=w360:dbl[][])
            n106 = Bundle By Name(cluster=w359, "Data set"=dbl[][] []) -> (w358:T15)
            n107 = call "Data set to SVM problem.vi"("Data set"=w360) -> ()  [unwired: 9 in, 2 out]
            n108 = Write to Text File(file (use dialog)=w353, text="", error in=w354) -> (refnum out=w351:refnum<file>, error out=w352:errorcluster)  [unwired: 1 in, 1 out]
            n109 = Close File(refnum=w351, error in=w352) -> (error out=w350:errorcluster)  [unwired: 1 out]
          }
          frame "SVM - Start predict" {
            w382 = T19 60 items=["MPU data"=42, "MPU data - DESCR"=43, "Accel calib parameters"=45, "Gyro calib parameters"=47, "Mag calib parameters - 1"=49, "Mag calib parameters - 2"=51, "YPR"=53, "YPR - DESCR"=54, "Strain sensors"=56, "Strain sensors - DESCR"=57, "Wristband"=59, "Wristband - DESCR"=60] ("BLE char handle")
            # "Needed to avoid double Check for event"
            n110 = Unbundle By Name(w378) -> ("Conn Status"=w381:T7)
            n111 = call "BLE - Enable notifications.vi"("Conn Status"=w381, "Descriptor handle"=w382, "Error In"=w379, "Enable notifications"=TRUE, "COM Bluegiga in"=w380) -> ("Error Out"=w377:errorcluster, "COM Bluegiga out"=w376:refnum<visa-resource-name>)  [unwired: 5 in]
            n112 = Flush Queue(queue=w374, error in (no error)=w375) -> (queue out=w385:refnum<queue>, error out=w384:errorcluster)  [unwired: 1 out]
            n113 = Wait (ms)(milliseconds to wait=u32 50) -> ()  [unwired: 1 out]
            n114 = Enqueue Element(queue=w385, element=SIENAR_Band_-_States."SVM - Check for event", error in (no error)=w384) -> ()  [unwired: 1 in, 3 out]
          }
          frame "Exit" {
          }
          frame "SVM - Load SVM model" {
            w399 = T11 {"param"={"svm_type"=enum."C_SVC", "kernel_type"=enum."LINEAR", "degree"=0, "gamma"=0.0, "coef0"=0.0, "cache_size"=0.0, "eps"=0.0, "C"=0.0, "weight_label"=[], "weight"=[], "nu"=0.0, "p"=0.0, "shrinking"=FALSE, "probability"=FALSE}, "nr_class"=0, "l"=0, "SV"=[], "sv_coef"=[], "rho"=[], "probA"=[], "probB"=[], "sv_indices"=[], "label"=[], "nSV"=[]}  # SVM Model
            # "#toDebug"
            n115 = call-poly <vilib>:"Read From XML File.vi"() -> ("error out"=w396:errorcluster, "XML Elements"=w397:string)  [unwired: 9 in, 1 out]
            n116 = Unflatten From XML(xml string=w397, type=w399, error in (no error)=w396) -> (value=w398:T11)  [unwired: 1 out]
            n117 = Bundle By Name(cluster=w401, "Model"=w398) -> (w400:T15)
          }
          frame "SVM - Save SVM model" {
            # "#toDebug"
            n118 = Unbundle By Name(w408) -> ("Model"=w407:T11)
            n119 = Flatten To XML(anything=w407) -> (xml string=w406:string)
            n120 = call-poly <vilib>:"Write to XML File.vi"("XML Input"=w406) -> ()  [unwired: 8 in, 3 out]
          }
        }
      }
      frame Error {
        n121 = Unbundle By Name(w419) -> ("code"=w421:i32)
        n122 = case shown="390" w421 {
          tunnel: [FALSE _ TRUE _ TRUE] -> w420
          tunnel: w419 -> [_ _ w427 w431 _]
          tunnel: [_ _ w427 _ _] -> w418
          tunnel: w417 -> [w424 w426 w428 w432 w448]
          tunnel: [w424 w426 w428 w430 w448] -> w416
          frame -1073807346 {
            n123 = One Button Dialog(message="The port selected for the connection with the BLED112\nis invalid. Please check and retry") -> ()  [unwired: 1 in, 1 out]
          }
          frame -1073807339 {
            n124 = One Button Dialog(message="Timeout event on serial port") -> ()  [unwired: 1 in, 1 out]
          }
          frame 0, Default {
          }
          frame 390 {
            n125 = Two Button Dialog(message="Connection problem: \nconnection handle is not valid", 2:"Reset dongle" ("T button name (\"OK\")")) -> (T button?=w433:bool)  [unwired: 1 in]
            n126 = case shown="False" w433 {
              tunnel: w432 -> [w438 w443]
              tunnel: w431 -> [w437 _]
              tunnel: [w438 w441] -> w430
              tunnel: [w437 w442] -> _
              frame False {
                w436 = FALSE ("Connect BLE")
                n127 = property on="BLE Status" class="Bool (strict)"("Value"=w436) -> ()  [unwired: 2 in, 2 out]
                n128 = property on="Connect BLE" class="Bool (strict)"("Value"=w436) -> ()  [unwired: 2 in, 2 out]
              }
              frame True {
                w439 = FALSE ("Connect BLE")
                n129 = call <vilib>:"ble_reset_dongle_and_cnx.vi"("error in (no error)"=errorcluster {"status"=FALSE, "code"=0, "source"=""}, "COM Bluegiga in"=w443) -> ("error out"=w447:errorcluster, "COM Bluegiga out"=w446:refnum<visa-resource-name>)  [unwired: 8 in]
                n130 = call <vilib>:"ble_attach_dongle.vi"("error in (no error)"=w447, "COM Bluegiga in"=w446) -> ("error out"=w444:errorcluster, "COM Bluegiga out"=w445:refnum<visa-resource-name>)  [unwired: 8 in]
                n131 = property on="BLE Status" class="Bool (strict)"("Value"=w439) -> ()  [unwired: 2 in, 2 out]
                n132 = property on="Connect BLE" class="Bool (strict)"("Value"=w439) -> ()  [unwired: 2 in, 2 out]
                n133 = call <vilib>:"ble_dongle_info.vi"("error in (no error)"=w444, "COM Bluegiga in"=w445) -> ("error out"=w442:errorcluster, "COM Bluegiga out"=w441:refnum<visa-resource-name>)  [unwired: 7 in, 1 out]
              }
            }
          }
          frame 1122 {
            # "This error is generated because of the reference of queue is closed\n(ex. the control loop has quit). Clear the error and close this loop"
          }
        }
      }
    }
    n134 = call "All close.vi"("Close? (F)"=w34) -> ("Close"=w45:bool)  [unwired: 9 in, 1 out]
  }
  n135 = while {
    tunnel: w21 -> [w455]
    tunnel: [w454] -> w27
    shift-right: [w453] -> w28
    shift-left: w20 -> [w456]
    stop <- w451 stop-if-true
    n136 = event shown="[20] \"Stream data\": Value Change" {
      selector: _ -> [_ _ _ _ _ _ _ _ _ _ _ _ _ _ _ _ _ _ _ _ _ _ _ _ _]
      dyn-events: _ -> [_ _ _ _ _ _ _ _ _ _ _ _ _ _ _ _ _ _ _ _ _ _ _ _ _]
      timeout: 200 -> [_ _ _ _ _ _ _ _ _ _ _ _ _ _ _ _ _ _ _ _ _ _ _ _ _]
      tunnel: w456 -> [w458 w462 w467 w472 w477 w482 w487 w495 w499 w503 w507 w511 w513 w518 w522 w531 w535 w539 w544 w549 w558 w566 w571 w579 w586]
      tunnel: [w458 w460 w466 w471 w475 w481 w486 w495 w498 w502 w506 w510 w513 w517 w521 w530 w534 w538 w543 w548 w557 w565 w570 w578 w584] -> w453
      tunnel: w455 -> [w459 w463 w468 w473 w478 w483 w488 w494 w496 w501 w505 w509 w514 w519 w523 w532 w536 w541 w545 w550 w559 w567 w572 w580 w587]
      tunnel: [w459 w461 w465 w470 w476 w480 w485 w494 w496 w501 w505 w509 w514 w516 w520 w529 w533 w541 w542 w547 w556 w564 w569 w577 w587] -> w454
      tunnel: [_ _ _ _ _ _ _ _ _ _ _ _ TRUE _ _ _ _ _ _ _ _ _ _ _ _] -> w450
      event Timeout {
        n137 = event-data() -> ()  [unwired: 1 in, 1 out]
      }
      event "Load data set": Value Change {
        n138 = event-data() -> ()  [unwired: 1 in, 2 out]
        n139 = Enqueue Element(queue=w463, element=SIENAR_Band_-_States."SVM - Load data set", error in (no error)=w462) -> (queue out=w461:refnum<queue>, error out=w460:errorcluster)  [unwired: 1 in, 1 out]
      }
      event "Learn from data": Value Change {
        n140 = event-data() -> ()  [unwired: 1 in, 2 out]
        n141 = Enqueue Element(queue=w468, element=SIENAR_Band_-_States."SVM - Learn from data", error in (no error)=w467) -> (queue out=w465:refnum<queue>, error out=w466:errorcluster)  [unwired: 1 in, 1 out]
      }
      event "Save Data set": Value Change {
        n142 = event-data() -> ()  [unwired: 1 in, 2 out]
        n143 = Enqueue Element(queue=w473, element=SIENAR_Band_-_States."SVM - Save data set", error in (no error)=w472) -> (queue out=w470:refnum<queue>, error out=w471:errorcluster)  [unwired: 1 in, 1 out]
      }
      event "Predict": Value Change {
        n144 = event-data() -> ()  [unwired: 1 in, 2 out]
        n145 = Enqueue Element(queue=w478, element=SIENAR_Band_-_States."SVM - Start predict", error in (no error)=w477) -> (queue out=w476:refnum<queue>, error out=w475:errorcluster)  [unwired: 1 in, 1 out]
      }
      event "Load SVM model": Value Change {
        n146 = event-data() -> ()  [unwired: 1 in, 6 out]
        n147 = Enqueue Element(queue=w483, element=SIENAR_Band_-_States."SVM - Load SVM model", error in (no error)=w482) -> (queue out=w480:refnum<queue>, error out=w481:errorcluster)  [unwired: 1 in, 1 out]
      }
      event "Save SVM model": Value Change {
        n148 = event-data() -> ()  [unwired: 1 in, 1 out]
        n149 = Enqueue Element(queue=w488, element=SIENAR_Band_-_States."SVM - Save SVM model", error in (no error)=w487) -> (queue out=w485:refnum<queue>, error out=w486:errorcluster)  [unwired: 1 in, 1 out]
      }
      event "Devices": Double Click {
        n150 = event-data() -> ("Row"=w492:i32)  [unwired: 1 in]
        n151 = property on="Devices" class="MCListbox (strict)"() -> ("ItemNames"=w491:string[][])  [unwired: 2 in, 2 out]
        n152 = Index Array(array=w491, index (row)=w492, index (col)=2 ("disabled index (col)")) -> (element=w490:string)
        n153 = local write "MAC Address"(w490) -> ()
      }
      event "Connection panel": Value Change {
        n154 = event-data() -> ()  [unwired: 1 in, 1 out]
        n155 = property on="Tab Control" class="TabCtl (strict)"(error in=w499, "Value"=T1."Connection Panel" ("Tab Control")) -> (error out=w498:errorcluster)  [unwired: 1 in, 1 out]
      }
      event "Settings panel": Value Change {
        n156 = event-data() -> ()  [unwired: 1 in, 1 out]
        n157 = property on="Tab Control" class="TabCtl (strict)"(error in=w503, "Value"=T1."Acquire Settings" ("Tab Control")) -> (error out=w502:errorcluster)  [unwired: 1 in, 1 out]
      }
      event "SVM Train panel": Value Change {
        n158 = event-data() -> ()  [unwired: 1 in, 1 out]
        n159 = property on="Tab Control" class="TabCtl (strict)"(error in=w507, "Value"=T1."SVM Training" ("Tab Control")) -> (error out=w506:errorcluster)  [unwired: 1 in, 1 out]
      }
      event "SVM Analysis panel": Value Change {
        n160 = event-data() -> ()  [unwired: 1 in, 1 out]
        n161 = property on="Tab Control" class="TabCtl (strict)"(error in=w511, "Value"=T1."SVM Analysis" ("Tab Control")) -> (error out=w510:errorcluster)  [unwired: 1 in, 1 out]
      }
      event "Exit": Value Change {
        n162 = event-data() -> ()  [unwired: 1 in, 1 out]
      }
      event "Connect dongle": Value Change {
        n163 = event-data() -> ()  [unwired: 1 in, 1 out]
        n164 = Enqueue Element(queue=w519, element=SIENAR_Band_-_States."Connect Dongle", error in (no error)=w518) -> (queue out=w516:refnum<queue>, error out=w517:errorcluster)  [unwired: 1 in, 1 out]
      }
      event "Discover": Value Change {
        n165 = event-data() -> ()  [unwired: 1 in, 1 out]
        n166 = Enqueue Element(queue=w523, element=SIENAR_Band_-_States."Discover BLE", error in (no error)=w522) -> (queue out=w520:refnum<queue>, error out=w521:errorcluster)  [unwired: 1 in, 1 out]
      }
      event "Connect BLE": Value Change {
        n167 = event-data() -> ("NewVal"=w528:bool)  [unwired: 1 in]
        n168 = Select(t=SIENAR_Band_-_States."Connect BLE", s=w528, f=SIENAR_Band_-_States."Disconnect BLE") -> (s? t:f=w525:T16)
        n169 = Enqueue Element(queue=w532, element=w525, error in (no error)=w531) -> (queue out=w529:refnum<queue>, error out=w530:errorcluster)  [unwired: 1 in, 1 out]
      }
      event "Confirm settings": Value Change {
        n170 = event-data() -> ()  [unwired: 1 in, 1 out]
        n171 = Enqueue Element(queue=w536, element=SIENAR_Band_-_States."Confirm settings", error in (no error)=w535) -> (queue out=w533:refnum<queue>, error out=w534:errorcluster)  [unwired: 1 in, 1 out]
      }
      event "Show RAW data": Value Change {
        n172 = event-data() -> ()  [unwired: 1 in, 1 out]
        n173 = property on="Tab Control" class="TabCtl (strict)"(error in=w539, "Value"=T1."Show RAW data" ("Tab Control")) -> (error out=w538:errorcluster)  [unwired: 1 in, 1 out]
      }
      event "Open MPU panel", "Open MPU calib": Value Change {
        n174 = event-data() -> ()  [unwired: 1 in, 2 out]
        n175 = Enqueue Element(queue=w545, element=SIENAR_Band_-_States."Open MPU panel", error in (no error)=w544) -> (queue out=w542:refnum<queue>, error out=w543:errorcluster)  [unwired: 1 in, 1 out]
      }
      event "Open adv viewer": Value Change {
        n176 = event-data() -> ()  [unwired: 1 in, 1 out]
        n177 = Enqueue Element(queue=w550, element=SIENAR_Band_-_States."Open advanced viewer", error in (no error)=w549) -> (queue out=w547:refnum<queue>, error out=w548:errorcluster)  [unwired: 1 in, 1 out]
      }
      event "Stream data": Value Change {
        n178 = event-data() -> ("NewVal"=w555:bool)  [unwired: 1 in]
        n179 = Select(t=SIENAR_Band_-_States."Set Stream settings", s=w555, f=SIENAR_Band_-_States."Stop stream") -> (s? t:f=w554:T16)
        n180 = Enqueue Element(queue=w559, element=w554, error in (no error)=w558) -> (queue out=w556:refnum<queue>, error out=w557:errorcluster)  [unwired: 1 in, 1 out]
      }
      event "Train": Value Change {
        n181 = event-data() -> ("NewVal"=w563:bool)  [unwired: 1 in]
        n182 = Select(t=SIENAR_Band_-_States."SVM - Train", s=w563, f=SIENAR_Band_-_States."Stop stream") -> (s? t:f=w560:T16)
        n183 = Enqueue Element(queue=w567, element=w560, error in (no error)=w566) -> (queue out=w564:refnum<queue>, error out=w565:errorcluster)  [unwired: 1 in, 1 out]
      }
      event Value Change {
        n184 = event-data() -> ()  [unwired: 1 in, 4 out]
        n185 = local read "Train"() -> (w568:bool)
        n186 = Select(t=SIENAR_Band_-_States."SVM - Train", s=w568, f=SIENAR_Band_-_States."Idle") -> (s? t:f=w573:T16)
        n187 = Enqueue Element(queue=w572, element=w573, error in (no error)=w571) -> (queue out=w569:refnum<queue>, error out=w570:errorcluster)  [unwired: 1 in, 1 out]
        n188 = local write "Event Count"(u32 0 ("Event Count")) -> ()
      }
      event "Save RAW data": Value Change {
        n189 = event-data() -> ()  [unwired: 1 in, 1 out]
        n190 = Enqueue Element(queue=w580, element=SIENAR_Band_-_States."Save RAW data", error in (no error)=w579) -> (queue out=w577:refnum<queue>, error out=w578:errorcluster)  [unwired: 1 in, 1 out]
      }
      event "Clear Plot": Value Change {
        n191 = event-data() -> ()  [unwired: 1 in, 1 out]
        n192 = property on="Strain chart" class="WFChart (strict)"(error in=w586, "History Data"=T27 []) -> (error out=w585:errorcluster)  [unwired: 1 in, 1 out]
        n193 = property on="YPR chart" class="WFChart (strict)"(error in=w585, "History Data"=cluster{"Yaw":i16, "Pitch":i16, "Roll":i16}[] []) -> (error out=w584:errorcluster)  [unwired: 1 in, 1 out]
      }
    }
    n194 = Or(x=w453, y=w450) -> (x .or. y?=w452:bool)
    n195 = call "All close.vi"("Close? (F)"=w452) -> ("Close"=w451:bool)  [unwired: 9 in, 1 out]
  }
  n196 = Release Queue(queue=w5, error in (no error)=w4) -> ()  [unwired: 1 in, 3 out]
  n197 = Unbundle By Name(w10) -> ("Is Connected"=w9:bool, "Conn Status"=w8:T7)
  n198 = Release Queue(queue=w27, error in (no error)=w28) -> ()  [unwired: 1 in, 3 out]
  n199 = case shown="False" w9 {
    tunnel: w11 -> [w589 w594]
    tunnel: w12 -> [w588 w593]
    tunnel: [w589 w592] -> w14
    tunnel: [w588 w591] -> w13
    tunnel: w8 -> [_ w590]
    frame False {
    }
    frame True {
      n200 = call <vilib>:"ble_disconnect_device.vi"("Connection Status"=w590, "error in (no error)"=w593, "COM Bluegiga in"=w594) -> ("error out"=w591:errorcluster, "COM Bluegiga out"=w592:refnum<visa-resource-name>)  [unwired: 7 in]
    }
  }
  n201 = VISA Close(VISA resource name=w14, error in (no error)=w13) -> (error out=w15:errorcluster)
  n202 = disable-structure shown="Enabled" {
    disable-tunnel: w15 -> [w595 _]
    frame Enabled {
      n203 = call <vilib>:"Simple Error Handler.vi"("error in (no error)"=w595) -> ()  [unwired: 4 in, 5 out]
    }
    frame Disabled {
    }
  }
